vi "试剂容量设置UI.vi"() -> ()   [LabVIEW 2016, in "斯坦道总磷总氮.lvlib"]
panel:
  in  "试剂容量":T1 {"V 14" format="%.0f mL"; "V 13" format="%.0f mL"; "V 12" format="%.0f mL"; "V 11" format="%.0f mL"; "V 10" format="%.0f mL"; "V 9" format="%.0f mL"; "V 8" format="%.0f mL"; "V 7" format="%.0f mL"; "V 6" format="%.0f mL"; "V 5" format="%.0f mL"; "V 4" format="%.0f mL"; "V 3" format="%.0f mL"; "V 2" format="%.0f mL"; "V" format="%.0f mL"}
  in  "取消":bool
  in  "确认":bool
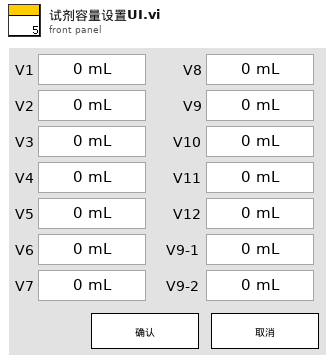
[diagram p1: front panel]
types:
  T1 = cluster{"V":u16, "V 2":u16, "V 3":u16, "V 4":u16, "V 5":u16, "V 6":u16, "V 7":u16, "V 8":u16, "V 9":u16, "V 10":u16, "V 11":u16, "V 12":u16, "V 13":u16, "V 14":u16}
  T2 = cluster{"时间标识":timestamp, "设备":string, "日志信息":string, "流程参数":string}
  T3 = cluster{"V1":sgl, "V2":sgl, "V3":sgl, "V4":sgl, "V5":sgl, "V6":sgl, "V7":sgl, "V8":sgl, "V9":sgl, "V10":sgl, "V11":sgl, "V12":sgl, "V9-1":sgl, "V9-2":sgl}
  T4 = cluster{"[0]":sgl, "[1]":sgl, "[2]":sgl, "[3]":sgl, "[4]":sgl, "[5]":sgl, "[6]":sgl, "[7]":sgl, "[8]":sgl, "[9]":sgl, "[10]":sgl, "[11]":sgl, "[12]":sgl, "[13]":sgl}
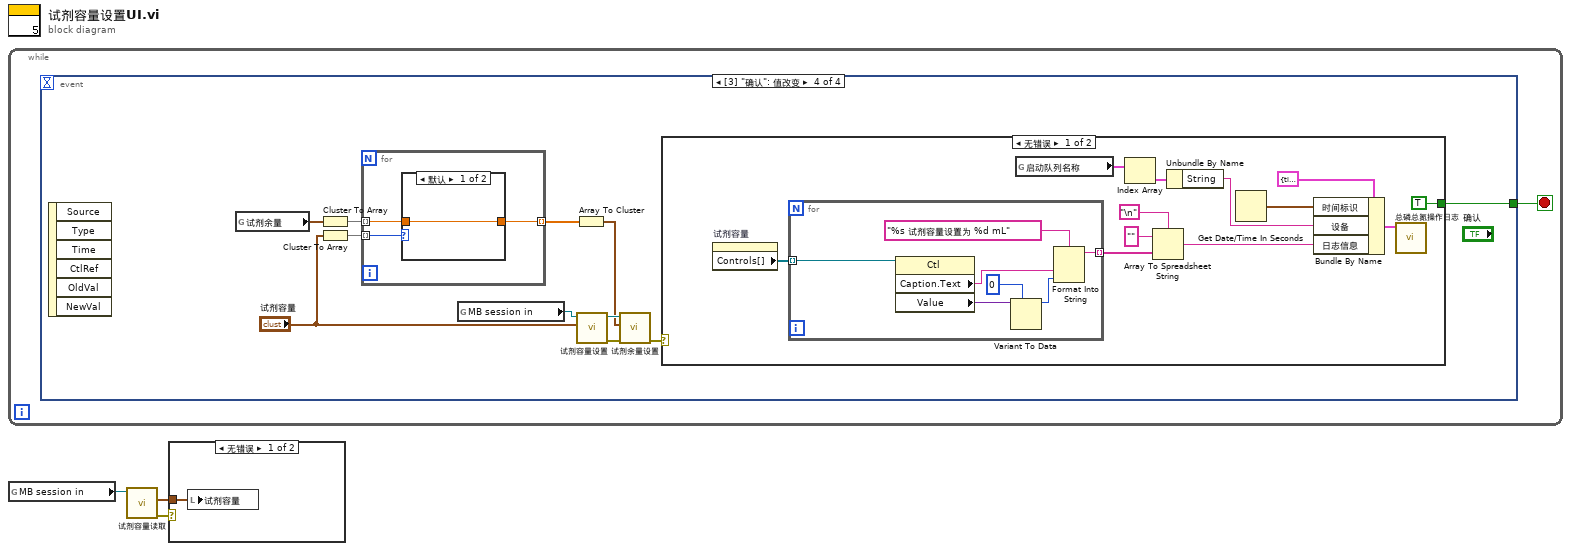
[diagram p0: block diagram]
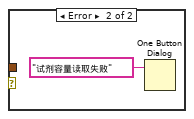
[diagram p2: hidden frame]
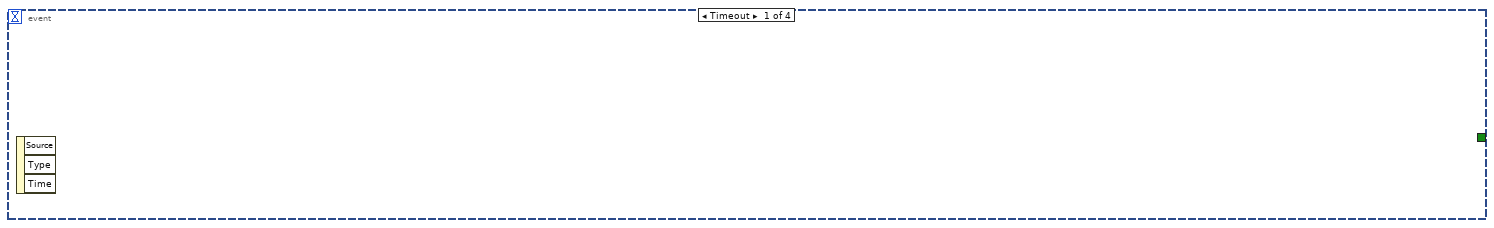
[diagram p3: hidden frame]
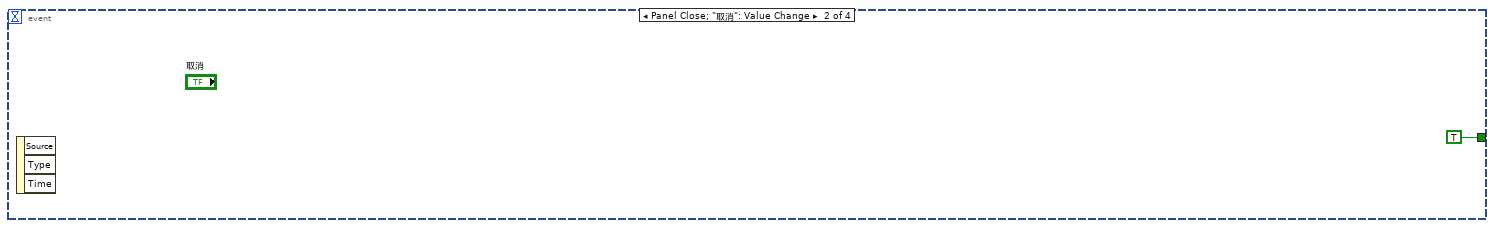
[diagram p4: hidden frame]
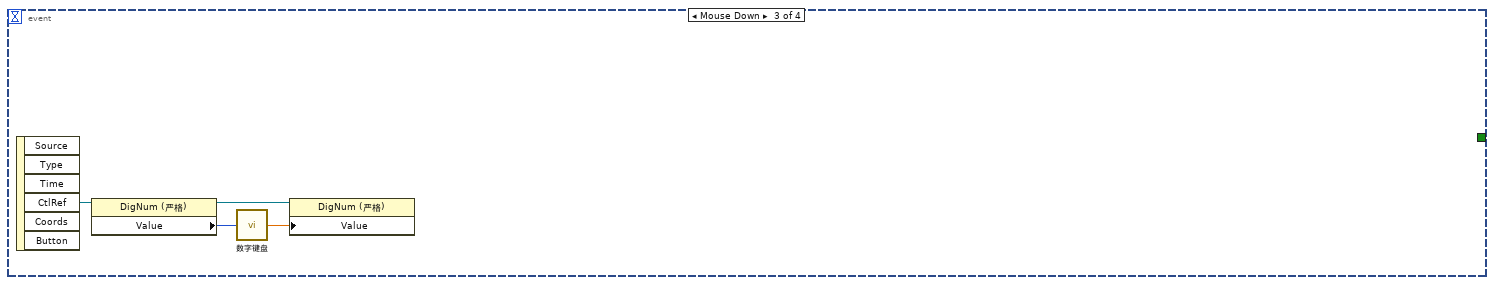
[diagram p5: hidden frame]
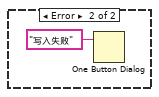
[diagram p7: hidden frame]
diagram:
  n1 = while {
    stop <- w4 stop-if-true
    n2 = event shown="[3] \"确认\": 值改变" {
      selector: _ -> [_ _ _ _]
      dyn-events: _ -> [_ _ _ _]
      timeout: _ -> [_ _ _ _]
      tunnel: [_ TRUE _ w20] -> w4
      event Timeout {
        n3 = event-data() -> ()  [unwired: 1 in, 3 out]
      }
      event Panel Close; "取消": Value Change {
        n4 = event-data() -> ()  [unwired: 1 in, 3 out]
      }
      event "试剂容量.V", "试剂容量.V 2", "试剂容量.V 3", "试剂容量.V 4", "试剂容量.V 5", "试剂容量.V 6", "试剂容量.V 7", "试剂容量.V 8", "试剂容量.V 9", "试剂容量.V 10", "试剂容量.V 11", "试剂容量.V 12", "试剂容量.V 13", "试剂容量.V 14": Mouse Down {
        n5 = event-data() -> ("CtlRef"=w9:refnum<vi>)  [unwired: 1 in, 5 out]
        n6 = property class="DigNum (严格)"(reference=w9) -> (reference out=w6:refnum<vi>, "Value"=w8:u16)  [unwired: 1 in, 1 out]
        n7 = call "数字键盘.vi"("OldNumber"=w8) -> ("NewNumber"=w7:dbl)
        n8 = property class="DigNum (严格)"(reference=w6, "Value"=w7) -> ()  [unwired: 1 in, 2 out]
      }
      event "确认": Value Change {
        n9 = event-data() -> ()  [unwired: 1 in, 6 out]
        n10 = global read "VAR总磷总氮全局变量.vi" "试剂余量"() -> (w14:T3)
        n11 = Cluster To Array(cluster=w14) -> (array=w12:sgl[])
        n12 = Cluster To Array(cluster="试剂容量") -> (array=w13:u16[])
        n13 = for {
          tunnel: w13 -> [w23] mode=indexing
          tunnel: w12 -> [w21] mode=indexing
          tunnel: [w22] -> w11 mode=indexing
          n14 = case shown="默认" w23 {
            tunnel: [w24 _] -> w22
            tunnel: w21 -> [w24 _]
            frame Default {
            }
            frame 0 {
            }
          }
        }
        n15 = global read "VAR总磷总氮全局变量.vi" "MB session in"() -> (w17:refnum<class "MB_Master.lvclass">)
        n16 = Array To Cluster(array=w11) -> (cluster=w10:T4)
        n17 = call "试剂容量设置.vi"("试剂容量"="试剂容量", "MB session in"=w17) -> ("error out"=w19:errorcluster, "MB session out"=w16:refnum<class "MB_Master.lvclass">)  [unwired: 8 in]
        n18 = call "试剂余量设置.vi"("Error in"=w19, "试剂余量"=w10, "MB session in"=w16) -> ("error out"=w18:errorcluster)  [unwired: 7 in, 1 out]
        n19 = case shown="无错误" w18 {
          tunnel: [TRUE _] -> w20
          frame No Error {
            n20 = property on="试剂容量" class="Clust (严格)"() -> ("Controls[]"=w31:refnum<vi>[])  [unwired: 2 in, 2 out]
            n21 = for {
              tunnel: w31 -> [w43] mode=indexing
              tunnel: [w37] -> w32 mode=indexing
              n22 = property class="Ctl"(reference=w43) -> ("Caption.Text"=w42:string, "Value"=w40:variant)  [unwired: 1 in, 2 out]
              n23 = Variant To Data(type=0, Variant=w40) -> (data=w38:i32)  [unwired: 1 in, 1 out]
              n24 = Format Into String(format string="%s 试剂容量设置为 %d mL" ("格式字符串"), w42, w38) -> (resulting string=w37:string)  [unwired: 2 in, 1 out]
            }
            n25 = global read "model config var.vi" "启动队列名称"() -> (w27:cluster{"String":string, "Value":u16}[])
            n26 = Index Array(array=w27) -> (element=w26:cluster{"String":string, "Value":u16})  [unwired: 1 in]
            n27 = Array To Spreadsheet String(delimiter (Tab)="\n", array=w32, 3:"" ("格式字符串")) -> (spreadsheet string=w34:string)
            n28 = Unbundle By Name(w26) -> ("String"=w25:string)
            n29 = Get Date/Time In Seconds() -> (seconds since 1Jan1904=w28:timestamp)
            n30 = Bundle By Name(cluster=T2 {"时间标识"=timestamp(0 s since 1904-01-01), "设备"="", "日志信息"="", "流程参数"=""} ("data in"), "时间标识"=w28, "设备"=w25, "日志信息"=w34) -> (w29:T2)
            n31 = call "总磷总氮操作日志.vi"("data in"=w29) -> ()  [unwired: 10 in, 1 out]
          }
          frame Error {
            n32 = One Button Dialog(message="写入失败" ("消息")) -> ()  [unwired: 1 in, 1 out]
          }
        }
      }
    }
  }
  n33 = global read "VAR总磷总氮全局变量.vi" "MB session in"() -> (w3:refnum<class "MB_Master.lvclass">)
  n34 = call "试剂容量读取.vi"("MB session in"=w3) -> ("error out"=w2:errorcluster, "试剂容量"=w1:T3)  [unwired: 8 in, 1 out]
  n35 = case shown="无错误" w2 {
    tunnel: w1 -> [w45 _]
    frame No Error {
      n36 = local write "试剂容量"(w45) -> ()
    }
    frame Error {
      n37 = One Button Dialog(message="试剂容量读取失败" ("消息")) -> ()  [unwired: 1 in, 1 out]
    }
  }
